vi "Begin.vi"(8 "error in":errorcluster, 11 "HARDWARE cluster":T7={"DRIVE MOTORS"=[], "Controller"=[], "ENCODERS"=[], "GYRO HARDWARE"={"Descr"="GYRO", "Installed?"=FALSE, "SPI Bus"=enum."SPI On-Board, CS0", "AnalogChannel"=enum."AI 0", "Calibrate On Open"=TRUE, "Calibrated Center Voltage"=0.0, "Calibration Time (s)"=2.0, "Sample Rate (Hz)"=100.0, "RefName"="", "stack name"="GYRO"}, "AIR"={"PRESSURE"=[], "COMPRESSOR"={"Descr"="COMPRESSOR", "Installed?"=TRUE, "Pneumatics Control Module"=0, "RefName"="COMPRESSOR", "stack name"="COMPRESSOR"}, "SOLENOIDS"=[]}, "MOTORS"=[], "SERVOS"=[], "SONAR"=[], "RELAY"=[], "LIMIT"=[]} {"MOTORS"."CAN ID" min=1 max=62 step=1; "MOTORS"."Motor Controller" items=["SPARK", "Existing", "SD540", "TALON SRX", "VICTOR SP", "TALON SR", "JAGUAR", "VICTOR"]; "AIR"."PRESSURE"."warning HIGH" format="%.2f"; "AIR"."PRESSURE"."warning LOW" format="%.2f"; "AIR"."PRESSURE"."nominal value" format="%.2f"; "DRIVE MOTORS"."CAN ID" min=1 max=62 step=1; "DRIVE MOTORS"."Motor Controller" items=["SPARK", "Existing", "SD540", "TALON SRX", "VICTOR SP", "TALON SR", "JAGUAR", "VICTOR"]; "Controller"."Parameters"."DEADBAND" format="%#_13g"; "Controller"."Parameters"."MIN SPEED" format="%#_13g"; "Controller"."Parameters"."MAX LIMIT" format="%#_13g"}) -> (0 "error out":errorcluster)   [LabVIEW 2019]
doc: "Called before other user functions, this VI is expected to open initial I/O refnums, load in file data, and do all program initialization. Notice that the <B>error out</B> terminal is simply used for data flow. Wiring it to other structures or subVIs ensures that this VI runs first."
uses:
  Controls/def HARDWARE CTRL info.ctl
  Controls/def MOTOR info.ctl
  Controls/ctrl MOTOR CTRLR SELECT.ctl
  <vilib>/Rock Robotics/SystemInterfaces/DIO/FPGA_DIOPWMChannel.ctl
  <vilib>/Rock Robotics/WPI/ThirdParty/REV Robotics/SPARK MAX/Typedef/Spark MAX Motor Type.ctl
  Controls/def USER CONTROL info.ctl
  <vilib>/Rock Robotics/WPI/Joystick/WPI_JoystickDeviceEnum.ctl
  Controls/def JOYSTICK PARAMETERS.ctl
  Controls/def ENCODER info.ctl
  <vilib>/Rock Robotics/SystemInterfaces/DIO/FPGA_DIOChannel.ctl
  <vilib>/Rock Robotics/WPI/Encoder/WPI_EncoderType.ctl
  Controls/def GYRO info.ctl
  <vilib>/Rock Robotics/SystemInterfaces/spilib/spi_bus.ctl
  Controls/ctrl ANALOG CHANNEL SELECT.ctl
  Controls/def AIR PRESSURE info.ctl
  <vilib>/Rock Robotics/SystemInterfaces/AI/FPGA_AIChannel.ctl
  Controls/def COMPRESSOR info.ctl
  Controls/def SOLENOID info.ctl
  <vilib>/Rock Robotics/WPI/Solenoid/WPI_SolenoidChannel.ctl
  <vilib>/Rock Robotics/WPI/Solenoid/WPI_SolenoidValue.ctl
  Controls/def SERVO info.ctl
  Controls/def SONAR info.ctl
  Controls/ctrl SONAR DEVICE SELECT.ctl
  <vilib>/Rock Robotics/WPI/Ultrasonic/WPI_UltrasonicRangeUnits.ctl
  Controls/def RELAY info.ctl
  <vilib>/Rock Robotics/SystemInterfaces/DIO/FPGA_DIORelayChannel.ctl
  <vilib>/Rock Robotics/WPI/Relay/WPI_RelayDirection.ctl
  <vilib>/Rock Robotics/WPI/Relay/WPI_RelayValue.ctl
  Controls/def LIMIT SWITCH info.ctl
  <vilib>/Rock Robotics/WPI/RobotDrive/WPI_RobotDriveDevRef.ctl
  <vilib>/Rock Robotics/WPI/MotorControl/WPI_MotorControlDeviceRef.ctl
  <vilib>/Rock Robotics/WPI/MotorControl/WPI_MotorControlType.ctl
  <vilib>/Rock Robotics/WPI/PWM/WPI_PWMDeadband.ctl
  <vilib>/Rock Robotics/WPI/DriverStation/WPI_DriverStationRobotMode2.ctl
  <vilib>/Rock Robotics/WPI/SafetyOutput/WPI_SafetyOutputConfigMenu.ctl
  Robot Global Data.vi
  <vilib>/Rock Robotics/WPI/Switch/WPI_SwitchOpenLimit.vi
  <vilib>/Rock Robotics/WPI/Solenoid/WPI_SolenoidOpenDouble.vi
  <vilib>/Rock Robotics/WPI/Solenoid/WPI_SolenoidOpenSingle.vi
  <vilib>/Rock Robotics/WPI/Solenoid/WPI_SolenoidSetEnum.vi
  <vilib>/Rock Robotics/WPI/Utilities/WPI_GetSetVariantRefNum.vi
  <vilib>/Rock Robotics/WPI/Counter/WPI_CounterDigitalInputToDigitalSource.vi
  <vilib>/Rock Robotics/WPI/MotorControl/WPI_MotorControlOpen SPARK.vi
  <vilib>/Rock Robotics/WPI/MotorControl/WPI_MotorControlOpen SD540.vi
  <vilib>/Rock Robotics/WPI/MotorControl/WPI_MotorControlOpen TalonSRX.vi
  <vilib>/Rock Robotics/WPI/MotorControl/WPI_MotorControlOpen VictorSP.vi
  <vilib>/Rock Robotics/WPI/MotorControl/WPI_MotorControlOpen Talon.vi
  <vilib>/Rock Robotics/WPI/MotorControl/WPI_MotorControlOpen Jaguar.vi
  <vilib>/Rock Robotics/WPI/MotorControl/WPI_MotorControlOpen Victor.vi
  Global  HARDWARE.vi
  <vilib>/Rock Robotics/WPI/Ultrasonic/WPI_SonarSRF08DeviceAddress.ctl
  <vilib>/Rock Robotics/SystemInterfaces/i2clib/i2c_bus.ctl
  <vilib>/Rock Robotics/WPI/Ultrasonic/WPI_SonarSRF04DigitalOpen.vi
  <vilib>/Rock Robotics/WPI/Ultrasonic/WPI_SonarSRF04DigitalRefNum Registry Set.vi
  <vilib>/Rock Robotics/WPI/Gyro/WPI_GyroAnalogOpen.vi
panel:
  out "RobotDriveDevRef":T1={"DevStatus"={"status"=FALSE, "code"=0, "source"=""}, "Motors[]"=[], "Square Inputs"=FALSE, "Max Output"=1.0}
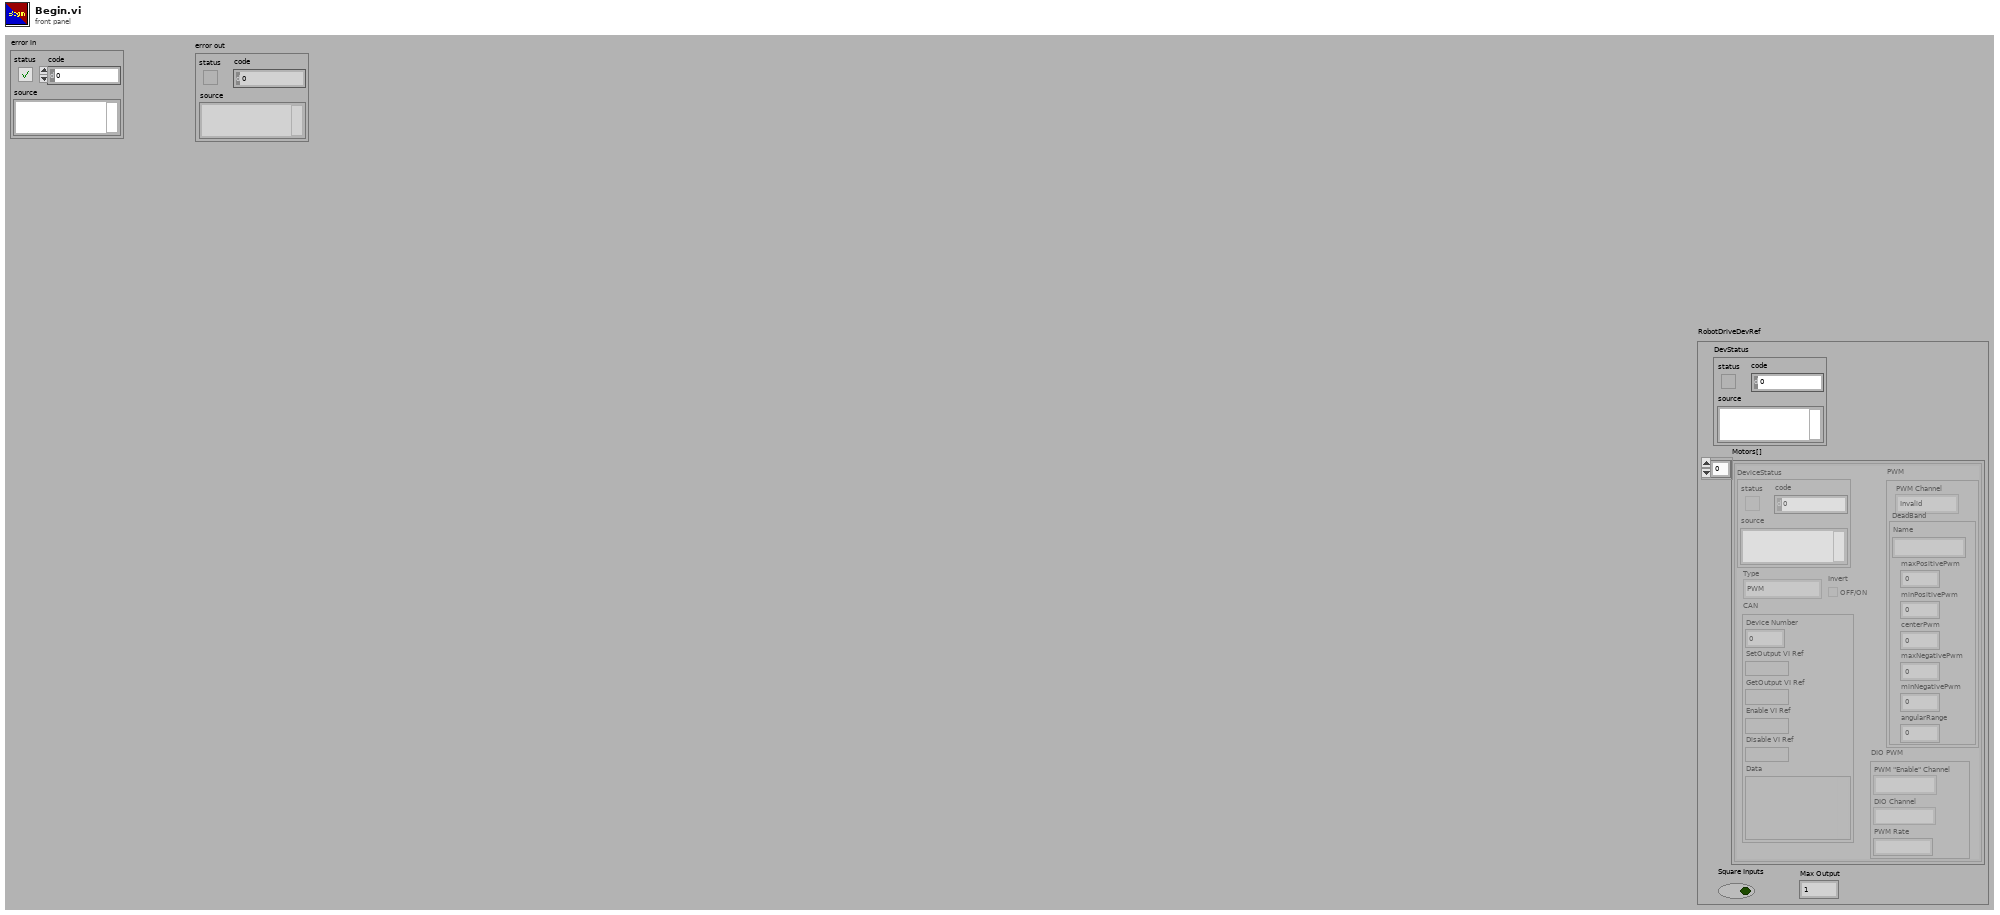
[diagram p1: front panel]
types:
  T1 = typedef "WPI_RobotDriveDevRef.ctl" = cluster{"DevStatus":errorcluster, "Motors[]":T2[], "Square Inputs":bool, "Max Output":dbl}
  T2 = typedef "WPI_MotorControlDeviceRef.ctl" = cluster{"DeviceStatus":errorcluster, "Type":T3, "PWM":cluster{"PWM Channel":T4, "DeadBand":T5}, "CAN":cluster{"Device Number":u8, "SetOutput VI Ref":variant, "GetOutput VI Ref":variant, "Enable VI Ref":variant, "Disable VI Ref":variant, "Data":variant}, "Invert":bool, "DIO PWM":cluster{"PWM \"Enable\" Channel":T4, "DIOChannel":T6, "PWM Rate":dbl}}
  T3 = typedef "WPI_MotorControlType.ctl" = enum16{"PWM", "CAN", "DIO PWM"}
  T4 = typedef "FPGA_DIOPWMChannel.ctl" = enum8{"PWM 0", "PWM 1", "PWM 2", "PWM 3", "PWM 4", "PWM 5", "PWM 6", "PWM 7", "PWM 8", "PWM 9", "PWM MXP 0", "PWM MXP 1", "PWM MXP 2", "PWM MXP 3", "PWM MXP 4", "PWM MXP 5", "PWM MXP 6", "PWM MXP 7", "PWM MXP 8", "PWM MXP 9", "Invalid"}
  T5 = typedef "WPI_PWMDeadband.ctl" = cluster{"Name":string, "maxPositivePwm":i32, "minPositivePwm":i32, "centerPwm":i32, "maxNegativePwm":i32, "minNegativePwm":i32, "angularRange":u16}
  T6 = typedef "FPGA_DIOChannel.ctl" = enum8{"DIO 0", "DIO 1", "DIO 2", "DIO 3", "DIO 4", "DIO 5", "DIO 6", "DIO 7", "DIO 8", "DIO 9", "DIO MXP 0", "DIO MXP 1", "DIO MXP 2", "DIO MXP 3", "DIO MXP 4", "DIO MXP 5", "DIO MXP 6", "DIO MXP 7", "DIO MXP 8", "DIO MXP 9", "DIO MXP 10", "DIO MXP 11", "DIO MXP 12", "DIO MXP 13", "DIO MXP 14", "DIO MXP 15", "SPI Port CS1", "SPI Port CS2", "SPI Port CS3", "SPI Port MISO", "SPI Port MOSI", "Invalid"}
  T7 = typedef "def HARDWARE CTRL info.ctl" = cluster{"DRIVE MOTORS":T8[], "Controller":T11[], "ENCODERS":T14[], "GYRO HARDWARE":T16, "AIR":cluster{"PRESSURE":T19[], "COMPRESSOR":T21, "SOLENOIDS":T22[]}, "MOTORS":T8[], "SERVOS":T25[], "SONAR":T26[], "RELAY":T29[], "LIMIT":T33[]}
  T8 = typedef "def MOTOR info.ctl" = cluster{"Descr":string, "Motor Controller":T9, "PWM ch":T4, "Invert?":bool, "Installed?":bool, "RefName":string, "stack name":string, "remove deadband":bool, "CAN ID":u8, "IDLE BEHAVIOUR":string, "Motor Type":T10}
  T9 = typedef "ctrl MOTOR CTRLR SELECT.ctl" = u16
  T10 = typedef "Spark MAX Motor Type.ctl" = enum16{"Brushed", "Brushless"}
  T11 = typedef "def USER CONTROL info.ctl" = cluster{"Descr":string, "Installed?":bool, "RefName":string, "JoystickDevice":T12, "Invert Y axis":bool, "Scale":dbl, "AXIS":string, "BUTTONS":string, "POV":string, "Parameters":T13}
  T12 = typedef "WPI_JoystickDeviceEnum.ctl" = enum16{"USB 0", "USB 1", "USB 2", "USB 3", "USB 4", "USB 5"}
  T13 = typedef "def JOYSTICK PARAMETERS.ctl" = cluster{"MAX LIMIT":dbl, "MIN SPEED":dbl, "DEADBAND":dbl, "invert X?":bool, "invert Y?":bool}
  T14 = typedef "def ENCODER info.ctl" = cluster{"Descr":string, "Installed?":bool, "A Channel":T6, "B Channel":T6, "Invert Direction":bool, "Enum":T15, "Gear ratio":dbl, "Cycles per Rev":dbl, "Diameter (in)":dbl[unit], "RefName":string, "stack name":string, "min rate (hz)":dbl, "Samples":u8, "STACK subnames":cluster{"RESET name":string, "STOPPED name":string, "DIRECTION name":string, "RATE name":string, "INSTALLED name":string}}
  T15 = typedef "WPI_EncoderType.ctl" = enum16{"1x", "2x", "4x"}
  T16 = typedef "def GYRO info.ctl" = cluster{"Descr":string, "Installed?":bool, "SPI Bus":T17, "AnalogChannel":T18, "Calibrate On Open":bool, "Calibrated Center Voltage":dbl, "Calibration Time (s)":dbl, "Sample Rate (Hz)":dbl, "RefName":string, "stack name":string}
  T17 = typedef "spi_bus.ctl" = enum16{"SPI On-Board, CS0", "SPI On-Board, CS1", "SPI On-Board, CS2", "SPI On-Board, CS3", "SPI MXP", "Invalid"}
  T18 = typedef "ctrl ANALOG CHANNEL SELECT.ctl" = enum8{"AI 0", "AI 1", "Invalid"}
  T19 = typedef "def AIR PRESSURE info.ctl" = cluster{"Descr":string, "Installed?":bool, "Channel":T20, "RefName":string, "stack name":string, "MULTIPLIER":dbl, "OFFSET":dbl, "nominal value":dbl, "warning LOW":dbl, "warning HIGH":dbl}
  T20 = typedef "FPGA_AIChannel.ctl" = enum8{"AI 0", "AI 1", "AI 2", "AI 3", "AI MXP 0", "AI MXP 1", "AI MXP 2", "AI MXP 3", "Invalid"}
  T21 = typedef "def COMPRESSOR info.ctl" = cluster{"Descr":string, "Installed?":bool, "Pneumatics Control Module":u8, "RefName":string, "stack name":string}
  T22 = typedef "def SOLENOID info.ctl" = cluster{"Descr":string, "Installed?":bool, "Pneumatics Control Module (0)":u8, "DBL":bool, "SolenoidChannel":T23, "SolenoidChannel":T23, "Default SET":T24, "RefName":string, "Value":string}
  T23 = typedef "WPI_SolenoidChannel.ctl" = enum8{"Solenoid 0", "Solenoid 1", "Solenoid 2", "Solenoid 3", "Solenoid 4", "Solenoid 5", "Solenoid 6", "Solenoid 7", "Invalid"}
  T24 = typedef "WPI_SolenoidValue.ctl" = enum16{"Off", "On", "Forward", "Reverse"}
  T25 = typedef "def SERVO info.ctl" = cluster{"Descr":string, "PWM ch":T4, "Installed?":bool, "Angular range":dbl, "RefName":string, "stack name":string}
  T26 = typedef "def SONAR info.ctl" = cluster{"Descr":string, "Installed?":bool, "Device type":T27, "PING Channel":T6, "ECHO Channel":T6, "RefName":string, "stack name":string, "Samples":i32, "Range Units":T28}
  T27 = typedef "ctrl SONAR DEVICE SELECT.ctl" = enum16{"SRF04 Digital", "MB1010 Digital", "MB1010 Analog", "SRF08 Digital"}
  T28 = typedef "WPI_UltrasonicRangeUnits.ctl" = enum16{"inches", "mm"}
  T29 = typedef "def RELAY info.ctl" = cluster{"Descr":string, "Installed?":bool, "RelayChannel":T30, "Relay Direction":T31, "Relay Value":T32, "RefName":string, "Value":string}
  T30 = typedef "FPGA_DIORelayChannel.ctl" = enum8{"Relay 0", "Relay 1", "Relay 2", "Relay 3", "Invalid"}
  T31 = typedef "WPI_RelayDirection.ctl" = enum16{"Both directions", "Forward only", "Reverse only"}
  T32 = typedef "WPI_RelayValue.ctl" = enum16{"Off", "On", "Forward", "Reverse"}
  T33 = typedef "def LIMIT SWITCH info.ctl" = cluster{"Descr":string, "Installed?":bool, "A Channel":T6, "Normally Closed?":bool, "RefName":string, "stack name":string}
  T34 = typedef "WPI_DriverStationRobotMode2.ctl" = enum16{"Autonomous Disabled", "Autonomous Enabled", "Teleop Disabled", "Teleop Enabled", "Disconnected", "Finish", "Test Disabled", "Test Enabled", "Emergency Stopped"}
  T35 = cluster{"PRESSURE":T19[], "COMPRESSOR":T21, "SOLENOIDS":T22[]}
  T36 = typedef "WPI_AnalogChannelDevRef.ctl" = cluster{"DevStatus":errorcluster, "Analog Channel":T20}
  T37 = typedef "WPI_SolenoidDevRef.ctl" = cluster{"DevStatus":errorcluster, "Pneumatics Control Module":u8, "Forward Solenoid Channel":T23, "Reverse Solenoid Channel":T23}
  T38 = typedef "WPI_CompressorDevRef.ctl" = cluster{"DevStatus":errorcluster, "Pneumatics Control Module":u8}
  T39 = typedef "WPI_RelayDevRef.ctl" = cluster{"DevStatus":errorcluster, "Relay Channel":T30, "Relay Direction":T31}
  T40 = typedef "WPI_SwitchDevRef.ctl" = cluster{"DevStatus":errorcluster, "DIO Channel":T6, "CntIndex":T41, "Normally Closed":bool}
  T41 = typedef "FPGA_CounterCtrSystemIndex.ctl" = enum8{"Ctr 0", "Ctr 1", "Ctr 2", "Ctr 3", "Ctr 4", "Ctr 5", "Ctr 6", "Ctr 7", "Invalid"}
  T42 = typedef "i2c_bus.ctl" = enum16{"I2C On-Board", "I2C MXP", "Invalid"}
  T43 = typedef "WPI_UltrasonicDeviceRef.ctl" = cluster{"DevStatus":errorcluster, "Ping Channel":T6, "Echo Channel":T6, "CntIndex":T41}
  T44 = typedef "WPI_SonarSRF08DeviceAddress.ctl" = u8
  T45 = typedef "WPI_ServoDeviceRef.ctl" = cluster{"DeviceStatus":errorcluster, "PWM Channel":T4, "DeadBand":T5}
  T46 = typedef "WPI_GyroDevRef.ctl" = cluster{"DevStatus":errorcluster, "Analog Channel":T20, "Gain (VoltsPerDegree/Second)":dbl, "Gyro Type":enum16{"Analog", "XRS450"}, "Handle":i32, "SPI Bus":T17, "Device Found":bool, "Sample Rate":dbl, "Calibrate On Open":bool, "Offset":dbl}
  T47 = typedef "WPI_JoystickDevRef.ctl" = cluster{"Device":T12}
  T48 = typedef "WPI_SafetyOutputConfigMenu.ctl" = enum16{"Enable", "Disable"}
  T49 = typedef "WPI_DigitalInputDevRef.ctl" = cluster{"DevStatus":errorcluster, "DIO Channel":T6}
  T50 = typedef "FPGA_CounterEncoderSourceConvertionLVSourceType.ctl" = cluster{"DevStatus":errorcluster, "AnalogTriggerMode?":bool, "DigitalMode":cluster{"DIO Channel":T51}, "AnalogTriggerMode":cluster{"AnalogTriggerIndex":T52, "OutputType":T53}}
  T51 = typedef "FPGA_DIODigitalSourceChannel.ctl" = enum8{"DIO 0", "DIO 1", "DIO 2", "DIO 3", "DIO 4", "DIO 5", "DIO 6", "DIO 7", "DIO 8", "DIO 9", "DIO MXP 0", "DIO MXP 1", "DIO MXP 2", "DIO MXP 3", "DIO MXP 4", "DIO MXP 5", "DIO MXP 6", "DIO MXP 7", "DIO MXP 8", "DIO MXP 9", "DIO MXP 10", "DIO MXP 11", "DIO MXP 12", "DIO MXP 13", "DIO MXP 14", "DIO MXP 15", "SPI Port CS1", "SPI Port CS2", "SPI Port CS3", "SPI Port MISO", "SPI Port MOSI", "Disabled"}
  T52 = typedef "FPGA_AnalogTriggerIndex.ctl" = enum8{"Trig 0", "Trig 1", "Trig 2", "Trig 3", "Trig 4", "Trig 5", "Trig 6", "Trig 7", "Invalid"}
  T53 = typedef "FPGA_AnalogTriggerOutType.ctl" = enum16{"InWindow", "TriggerState", "Rising", "Falling"}
  T54 = typedef "WPI_EncoderDevRef.ctl" = cluster{"DevStatus":errorcluster, "EncoderIndex":T55, "CounterIndex":T41, "DistancePerCount":dbl, "Decoding Type":T15}
  T55 = typedef "FPGA_EncoderIdx.ctl" = enum8{"Enc 0", "Enc 1", "Enc 2", "Enc 3", "Enc 4", "Enc 5", "Enc 6", "Enc 7", "Invalid"}
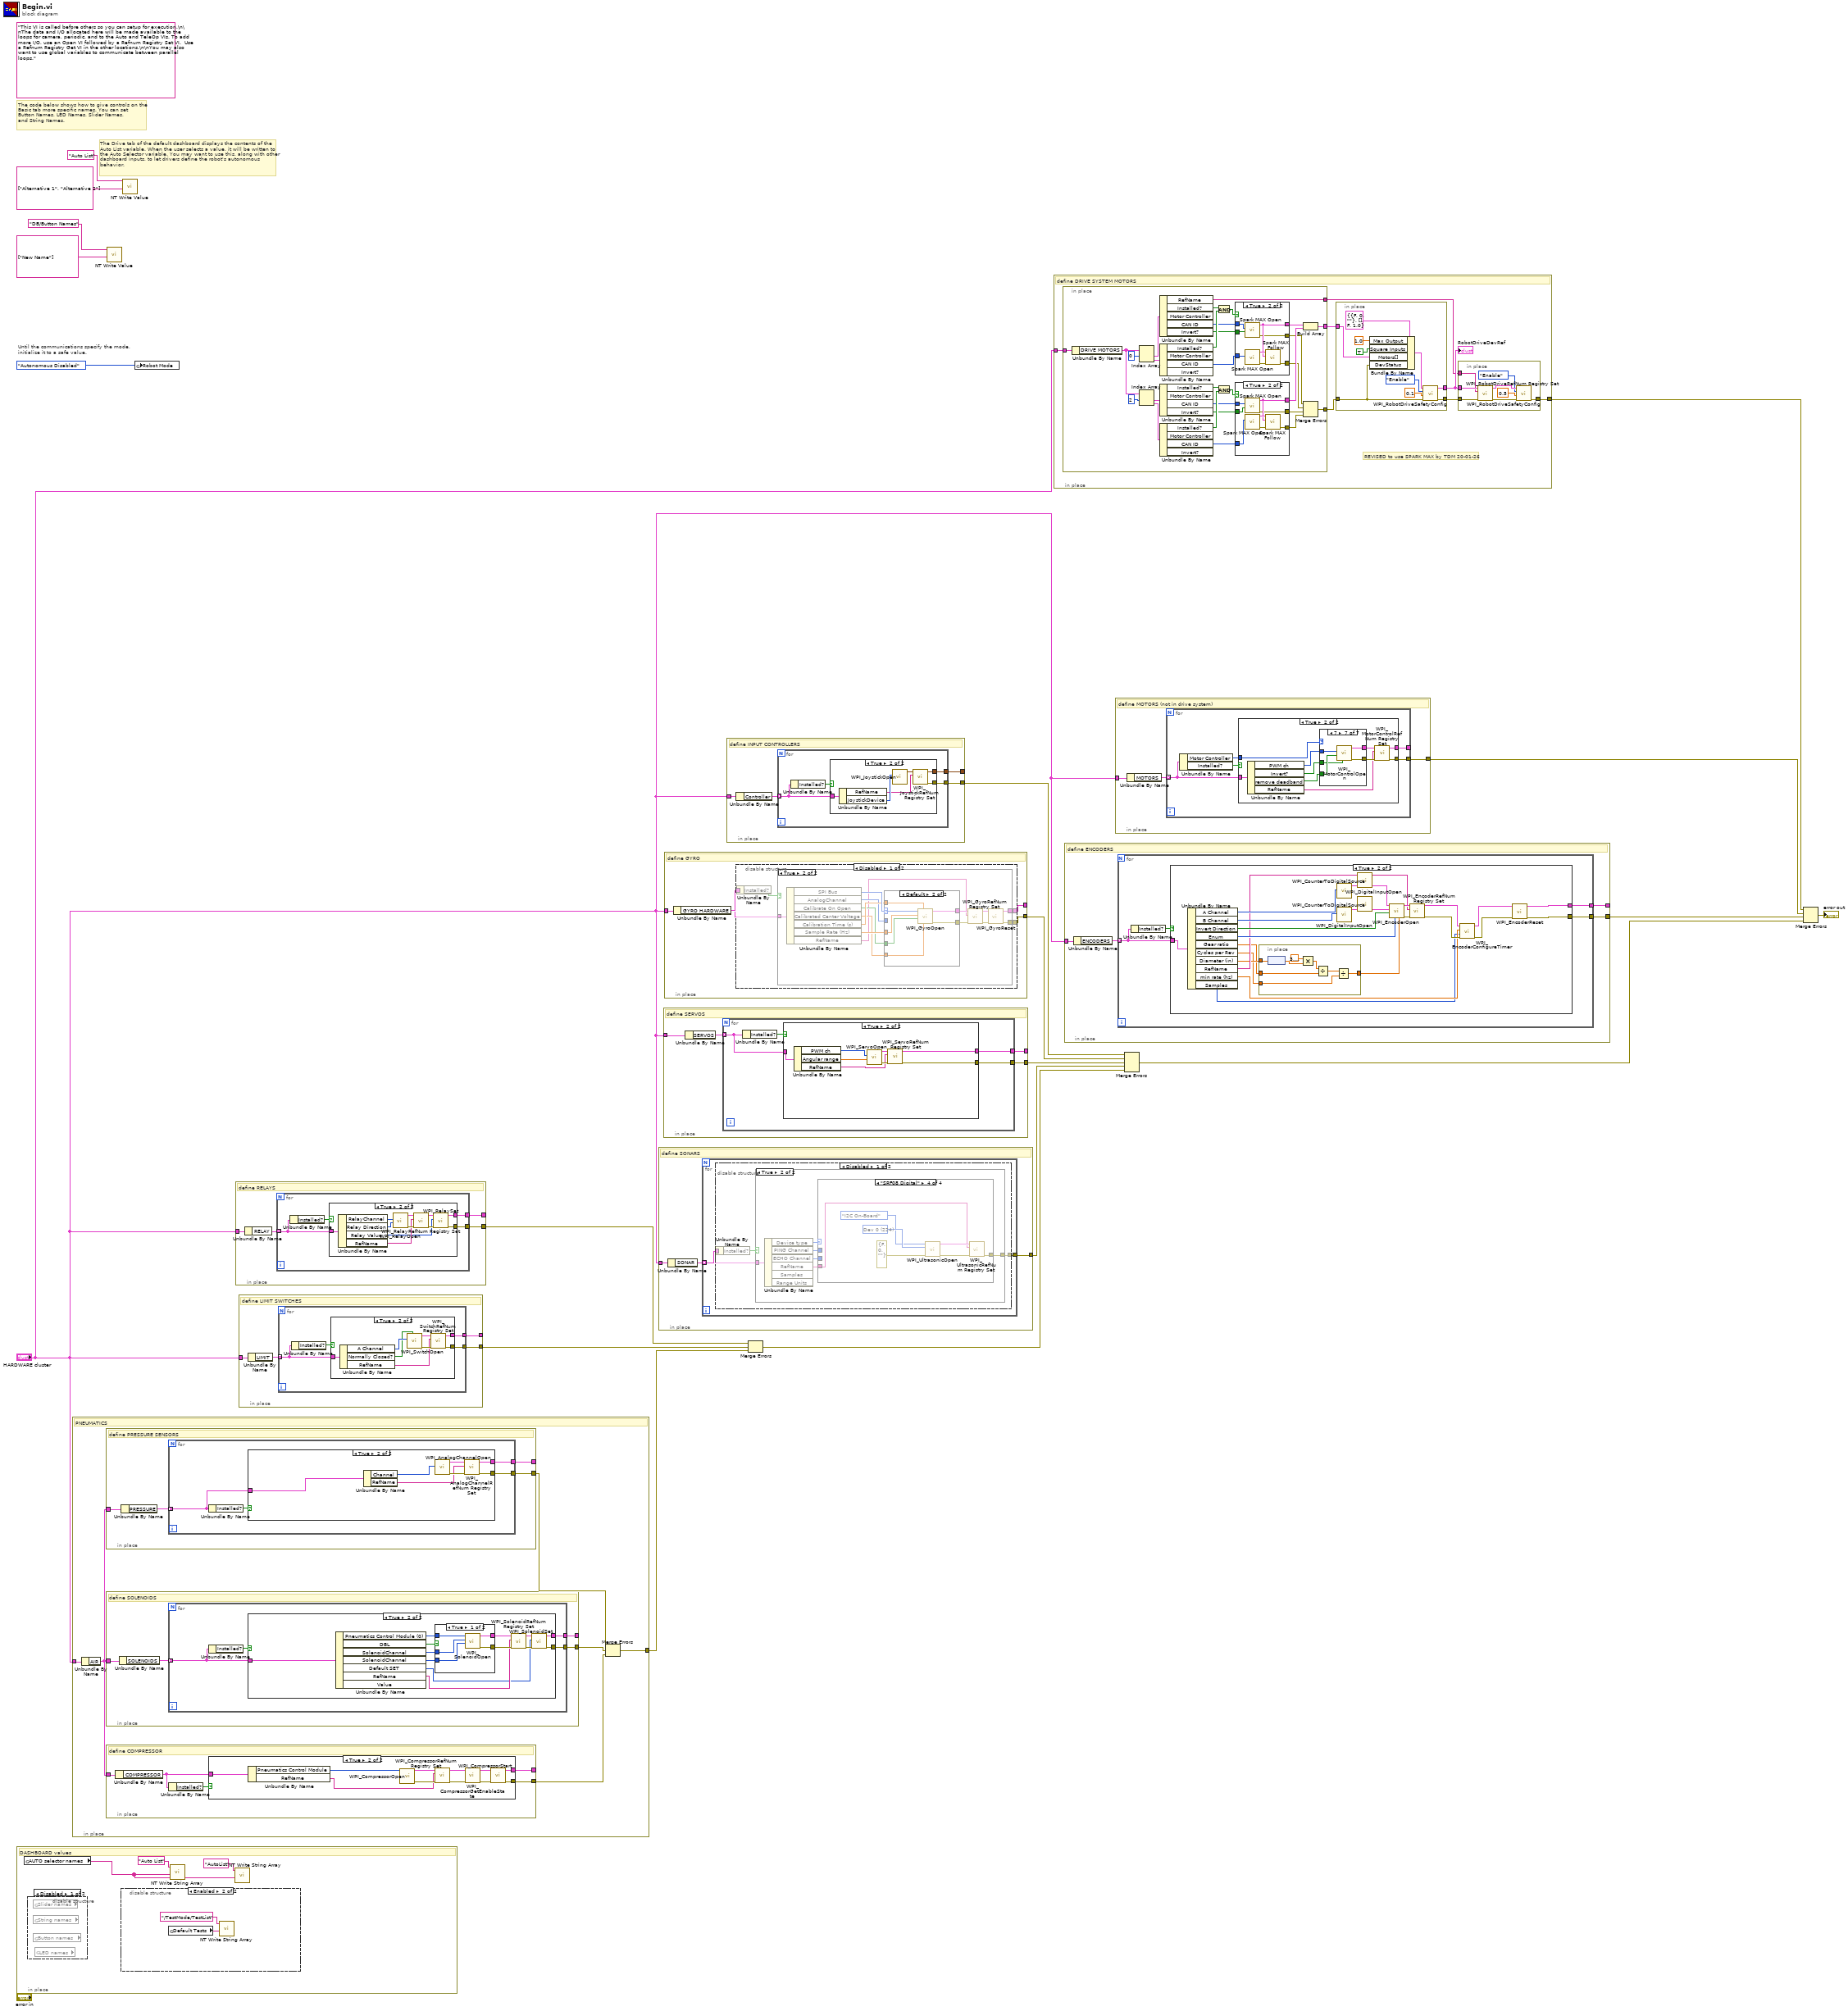
[diagram p0: block diagram]
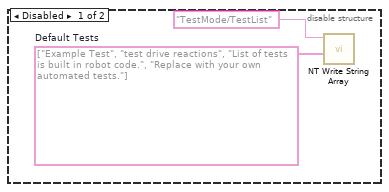
[diagram p2: hidden frame]
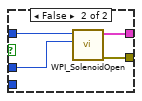
[diagram p6: hidden frame]
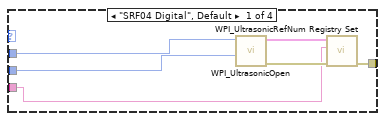
[diagram p11: hidden frame]
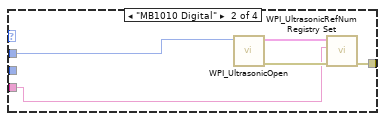
[diagram p12: hidden frame]
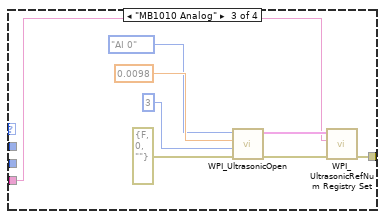
[diagram p13: hidden frame]
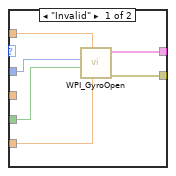
[diagram p17: hidden frame]
diagram:
  (unwired) "This VI is called before others so you can setup for execution.\n\nThe data and I/O allocated here will be made available to the loops for camera, periodic, and to the Auto and TeleOp VIs. To add more I/O, use an Open VI followed by a Refnum Registry Set VI.  Use a Refnum Registry Get VI in the other locations.\n\nYou may also want to use global variables to communicate between parallel loops."
  # "The Drive tab of the default dashboard displays the contents of the\nAuto List variable. When the user selects a value, it will be written to\nthe Auto Selector variable. You may want to use this, along with other\ndashboard inputs, to let drivers define the robot's autonomous\nbehavior."
  # "The code below shows how to give controls on the\nBasic tab more specific names. You can set\nButton Names, LED Names, Slider Names,\nand String Names."
  # "Until the communications specify the mode,\ninitialize it to a safe value."
  n1 = in-place {
    # "DASHBOARD values"
    n2 = global read "Global  HARDWARE.vi" "AUTO selector names"() -> (w20:string[])
    n3 = disable-structure shown="Disabled" {
      frame Disabled {
        n4 = global read "Global  HARDWARE.vi" "Slider names"() -> ()  [unwired: 1 out]
        n5 = global read "Global  HARDWARE.vi" "String names"() -> ()  [unwired: 1 out]
        n6 = global read "Global  HARDWARE.vi" "Button names"() -> ()  [unwired: 1 out]
        n7 = global read "Global  HARDWARE.vi" "LED names"() -> ()  [unwired: 1 out]
      }
      frame Enabled {
      }
    }
    n8 = disable-structure shown="Enabled" {
      frame Disabled {
        w24 = string[] ["Example Test", "test drive reactions", "List of tests is built in robot code.", "Replace with your own automated tests."]  # Default Tests
        n9 = call <vilib>:"NT Write String Array.vi"("String Array"=w24, "Name"="TestMode/TestList") -> ()  [unwired: 9 in, 1 out]
      }
      frame Enabled {
        n10 = global read "Global  HARDWARE.vi" "Default Tests"() -> (w26:string[])
        n11 = call <vilib>:"NT Write String Array.vi"("String Array"=w26, "Name"="/TestMode/TestList") -> ()  [unwired: 9 in, 1 out]
      }
    }
    n12 = call <vilib>:"NT Write String Array.vi"("String Array"=w20, "Name"="Auto List") -> ()  [unwired: 9 in, 1 out]
    n13 = call <vilib>:"NT Write String Array.vi"("String Array"=w20, "Name"="AutoList") -> ()  [unwired: 9 in, 1 out]
  }
  n14 = in-place {
    in-place-border: "HARDWARE cluster" -> [w32]
    in-place-border: [w27] -> w3
    # "PNEUMATICS"
    n15 = Unbundle By Name(w32) -> ("AIR"=w31:T35)
    n16 = in-place {
      in-place-border: w31 -> [w36]
      in-place-border: [w34] -> _
      in-place-border: [w33] -> w28
      # "define PRESSURE SENSORS"
      n17 = Unbundle By Name(w36) -> ("PRESSURE"=w35:T19[])
      n18 = for {
        tunnel: w35 -> [w39] mode=indexing
        tunnel: [w38] -> w34
        tunnel: [w37] -> w33
        n19 = Unbundle By Name(w39) -> ("Installed?"=w40:bool)
        n20 = case shown="True" w40 {
          tunnel: w39 -> [_ w47]
          tunnel: [_ w42] -> w38
          tunnel: [_ w41] -> w37
          frame False {
          }
          frame True {
            n21 = Unbundle By Name(w47) -> ("Channel"=w44:T20, "RefName"=w43:string)
            n22 = call <vilib>:"WPI_AnalogChannelOpen.vi"("Analog Channel"=w44) -> ("error out"=w45:errorcluster, "AIDeviceRef"=w46:T36)  [unwired: 9 in]
            n23 = call <vilib>:"WPI_AnalogChannelRefNum Registry Set.vi"("error in (no error)"=w45, "refnum name"=w43, "AIDeviceRef"=w46) -> ("error out"=w41:errorcluster, "AIDeviceRef"=w42:T36)  [unwired: 7 in]
          }
        }
      }
    }
    n24 = in-place {
      in-place-border: w31 -> [w51]
      in-place-border: [w49] -> _
      in-place-border: [w48] -> w29
      # "define SOLENOIDS"
      n25 = Unbundle By Name(w51) -> ("SOLENOIDS"=w50:T22[])
      n26 = for {
        tunnel: w50 -> [w54] mode=indexing
        tunnel: [w53] -> w49
        tunnel: [w52] -> w48
        n27 = Unbundle By Name(w54) -> ("Installed?"=w55:bool)
        n28 = case shown="True" w55 {
          tunnel: w54 -> [_ w68]
          tunnel: [_ w57] -> w53
          tunnel: [_ w56] -> w52
          frame False {
          }
          frame True {
            n29 = Unbundle By Name(w68) -> ("Pneumatics Control Module (0)"=w67:u8, "DBL"=w66:bool, "SolenoidChannel"=w65:T23, "SolenoidChannel"=w64:T23, "Default SET"=w58:T24, "RefName"=w62:string)  [unwired: 1 out]
            n30 = case shown="True" w66 {
              tunnel: w67 -> [w73 w77]
              tunnel: w65 -> [w72 w76]
              tunnel: w64 -> [w71 _]
              tunnel: [w70 w75] -> w61
              tunnel: [w69 w74] -> w63
              frame True {
                n31 = call-poly <vilib>:"WPI_SolenoidOpen.vi"("Reverse Solenoid Channel"=w71, "Forward Solenoid Channel"=w72, "Pneumatics Control Module (0)"=w73) -> ("error out"=w69:errorcluster, "SolenoidDevRef"=w70:T37)  [unwired: 7 in]
              }
              frame False {
                n32 = call-poly <vilib>:"WPI_SolenoidOpen.vi"("Solenoid Channel"=w76, "Pneumatics Control Module (0)"=w77) -> ("error out"=w74:errorcluster, "SolenoidDevRef"=w75:T37)  [unwired: 8 in]
              }
            }
            n33 = call <vilib>:"WPI_SolenoidRefNum Registry Set.vi"("error in (no error)"=w63, "refnum name"=w62, "SolenoidDevRef"=w61) -> ("error out"=w60:errorcluster, "SolenoidDevRef"=w59:T37)  [unwired: 7 in]
            n34 = call-poly <vilib>:"WPI_SolenoidSet.vi"("error in (no error)"=w60, "Value"=w58, "SolenoidDevRef"=w59) -> ("error out"=w56:errorcluster, "SolenoidDevRef"=w57:T37)  [unwired: 7 in]
          }
        }
      }
    }
    n35 = in-place {
      in-place-border: w31 -> [w82]
      in-place-border: [w79] -> _
      in-place-border: [w78] -> w30
      # "define COMPRESSOR"
      n36 = Unbundle By Name(w82) -> ("COMPRESSOR"=w80:T21)
      n37 = Unbundle By Name(w80) -> ("Installed?"=w81:bool)
      n38 = case shown="True" w81 {
        tunnel: w80 -> [_ w91]
        tunnel: [_ w84] -> w79
        tunnel: [_ w83] -> w78
        frame False {
        }
        frame True {
          n39 = Unbundle By Name(w91) -> ("Pneumatics Control Module"=w90:u8, "RefName"=w89:string)
          n40 = call <vilib>:"WPI_CompressorOpen.vi"("Pneumatics Control Module (0)"=w90) -> ("CompressorDevRef"=w92:T38, "error out"=w93:errorcluster)  [unwired: 13 in]
          n41 = call <vilib>:"WPI_CompressorRefNum Registry Set.vi"("error in (no error)"=w93, "refnum name"=w89, "CompressorDevRef"=w92) -> ("error out"=w88:errorcluster, "CompressorDevRef"=w87:T38)  [unwired: 7 in]
          n42 = call <vilib>:"WPI_CompressorGetEnableState.vi"("error in (no error)"=w88, "CompressorDevRef"=w87) -> ("error out"=w86:errorcluster, "CompressorDevRef"=w85:T38)  [unwired: 6 in, 2 out]
          n43 = call <vilib>:"WPI_CompressorStart.vi"("error in (no error)"=w86, "CompressorDevRef"=w85) -> ("error out"=w83:errorcluster, "CompressorDevRef"=w84:T38)  [unwired: 8 in]
        }
      }
    }
    n44 = Merge Errors(w28, w29, w30) -> (w27:errorcluster)
  }
  n45 = call-poly <vilib>:"NT Write Value.vi"("String Array"=string[] ["New Name"], "Name"="DB/Button Names") -> ()  [unwired: 9 in, 1 out]
  n46 = call-poly <vilib>:"NT Write Value.vi"("String Array"=string[] ["Alternative 1", "Alternative 2"], "Name"="Auto List") -> ()  [unwired: 9 in, 1 out]
  n47 = global write "Robot Global Data.vi" "Robot Mode"(WPI_DriverStationRobotMode2."Autonomous Disabled" ("Robot Mode")) -> ()
  n48 = in-place {
    in-place-border: "HARDWARE cluster" -> [w97]
    in-place-border: [w95] -> _
    in-place-border: [w94] -> w13
    # "define RELAYS"
    n49 = Unbundle By Name(w97) -> ("RELAY"=w96:T29[])
    n50 = for {
      tunnel: w96 -> [w100] mode=indexing
      tunnel: [w99] -> w95
      tunnel: [w98] -> w94
      n51 = Unbundle By Name(w100) -> ("Installed?"=w101:bool)
      n52 = case shown="True" w101 {
        tunnel: w100 -> [_ w110]
        tunnel: [_ w103] -> w99
        tunnel: [_ w102] -> w98
        frame False {
        }
        frame True {
          n53 = Unbundle By Name(w110) -> ("RelayChannel"=w109:T30, "Relay Direction"=w108:T31, "Relay Value"=w104:T32, "RefName"=w107:string)
          n54 = call <vilib>:"WPI_RelayOpen.vi"("Relay Direction"=w108, "Relay Channel"=w109) -> ("error out"=w112:errorcluster, "RelayDevRef"=w111:T39)  [unwired: 8 in]
          n55 = call <vilib>:"WPI_RelayRefNum Registry Set.vi"("error in (no error)"=w112, "refnum name"=w107, "RelayDevRef"=w111) -> ("error out"=w106:errorcluster, "RelayDevRef"=w105:T39)  [unwired: 7 in]
          n56 = call <vilib>:"WPI_RelaySet.vi"("error in (no error)"=w106, "RelayValue"=w104, "RelayDevRef"=w105) -> ("error out"=w102:errorcluster, "RelayDevRef"=w103:T39)  [unwired: 7 in]
        }
      }
    }
  }
  n57 = in-place {
    in-place-border: "HARDWARE cluster" -> [w116]
    in-place-border: [w114] -> _
    in-place-border: [w113] -> w12
    # "define LIMIT SWITCHES"
    n58 = Unbundle By Name(w116) -> ("LIMIT"=w115:T33[])
    n59 = for {
      tunnel: w115 -> [w119] mode=indexing
      tunnel: [w118] -> w114
      tunnel: [w117] -> w113
      n60 = Unbundle By Name(w119) -> ("Installed?"=w120:bool)
      n61 = case shown="True" w120 {
        tunnel: w119 -> [_ w128]
        tunnel: [_ w122] -> w118
        tunnel: [_ w121] -> w117
        frame False {
        }
        frame True {
          n62 = Unbundle By Name(w128) -> ("A Channel"=w127:T6, "Normally Closed?"=w126:bool, "RefName"=w123:string)
          n63 = call-poly <vilib>:"WPI_SwitchOpen.vi"("Normally Closed"=w126, "DIO Channel"=w127) -> ("error out"=w125:errorcluster, "SwitchDevRef"=w124:T40)  [unwired: 8 in]
          n64 = call <vilib>:"WPI_SwitchRefNum Registry Set.vi"("error in (no error)"=w125, "refnum name"=w123, "SwitchDevRef"=w124) -> ("error out"=w121:errorcluster, "SwitchDevRef"=w122:T40)  [unwired: 7 in]
        }
      }
    }
  }
  n65 = in-place {
    in-place-border: "HARDWARE cluster" -> [w131]
    in-place-border: [w129] -> w9
    # "define SONARS"
    n66 = Unbundle By Name(w131) -> ("SONAR"=w130:T26[])
    n67 = for {
      tunnel: w130 -> [w133] mode=indexing
      tunnel: [w132] -> w129
      n68 = disable-structure shown="Disabled" {
        disable-tunnel: w133 -> [w135 _]
        disable-tunnel: [w134 _] -> w132
        frame Disabled {
          n69 = Unbundle By Name(w135) -> ("Installed?"=w136:bool)
          n70 = case shown="True" w136 {
            tunnel: w135 -> [_ w142]
            tunnel: [_ w137] -> w134
            frame False {
            }
            frame True {
              n71 = Unbundle By Name(w142) -> ("Device type"=w139:T27, "PING Channel"=w141:T6, "ECHO Channel"=w140:T6, "RefName"=w138:string)  [unwired: 2 out]
              n72 = case shown="\"SRF08 Digital\"" w139 {
                tunnel: w141 -> [w148 w153 _ _]
                tunnel: w140 -> [w147 _ _ _]
                tunnel: w138 -> [w145 w149 w154 w162]
                tunnel: [w143 w151 w157 w164] -> w137
                frame "SRF04 Digital", Default {
                  n73 = call-poly <vilib>:"WPI_UltrasonicOpen.vi"("Echo DIO Channel"=w147, "Ping DIO Channel"=w148) -> ("error out"=w146:errorcluster, "SonarSRF04DevRef"=w144:T43)  [unwired: 8 in]
                  n74 = call-poly <vilib>:"WPI_UltrasonicRefNum Registry Set.vi"("error in (no error)"=w146, "refnum name"=w145, "SonarSRF04DevRef"=w144) -> ("error out"=w143:errorcluster)  [unwired: 7 in, 1 out]
                }
                frame "MB1010 Digital" {
                  n75 = call-poly <vilib>:"WPI_UltrasonicOpen.vi"("Ping DIO Channel"=w153) -> ("error out"=w152:errorcluster, "SonarSRF04DevRef"=w150:T43)  [unwired: 9 in]
                  n76 = call-poly <vilib>:"WPI_UltrasonicRefNum Registry Set.vi"("error in (no error)"=w152, "refnum name"=w149, "SonarSRF04DevRef"=w150) -> ("error out"=w151:errorcluster)  [unwired: 7 in, 1 out]
                }
                frame "MB1010 Analog" {
                  n77 = call-poly <vilib>:"WPI_UltrasonicOpen.vi"("error in (no error)"=errorcluster {"status"=FALSE, "code"=0, "source"=""} ("error in"), "Echo DIO Channel"=u8 3 ("Average Bits"), 10:0.0098 ("Scaling factor (V/in)"), "Ping DIO Channel"=FPGA_AIChannel."AI 0" ("Analog Channel")) -> ("error out"=w156:errorcluster, "SonarSRF04DevRef"=w155:T43)  [unwired: 6 in]
                  n78 = call-poly <vilib>:"WPI_UltrasonicRefNum Registry Set.vi"("error in (no error)"=w156, "refnum name"=w154, "SonarSRF04DevRef"=w155) -> ("error out"=w157:errorcluster)  [unwired: 7 in, 1 out]
                }
                frame "SRF08 Digital" {
                  w167 = T44 224 items=["Dev 0"=224, "Dev 1"=226, "Dev 2"=228, "Dev 3"=230, "Dev 4"=232, "Dev 5"=234, "Dev 6"=236, "Dev 7"=238, "Dev 8"=240, "Dev 9"=242, "Dev 10"=244, "Dev 11"=246, "Dev 12"=248, "Dev 13"=250, "Dev 14"=252, "Dev 15"=254] ("Device Address")
                  n79 = call-poly <vilib>:"WPI_UltrasonicOpen.vi"("error in (no error)"=errorcluster {"status"=FALSE, "code"=0, "source"=""} ("error in"), 10:w167, "Ping DIO Channel"=i2c_bus."I2C On-Board" ("I2C Bus")) -> ("error out"=w163:errorcluster, "SonarSRF04DevRef"=w165:T43)  [unwired: 7 in]
                  n80 = call-poly <vilib>:"WPI_UltrasonicRefNum Registry Set.vi"("error in (no error)"=w163, "refnum name"=w162, "SonarSRF04DevRef"=w165) -> ("error out"=w164:errorcluster)  [unwired: 7 in, 1 out]
                }
              }
            }
          }
        }
        frame Enabled {
        }
      }
    }
  }
  n81 = in-place {
    in-place-border: "HARDWARE cluster" -> [w172]
    in-place-border: [w170] -> _
    in-place-border: [w169] -> w11
    # "define SERVOS"
    n82 = Unbundle By Name(w172) -> ("SERVOS"=w171:T25[])
    n83 = for {
      tunnel: w171 -> [w175] mode=indexing
      tunnel: [w174] -> w170
      tunnel: [w173] -> w169
      n84 = Unbundle By Name(w175) -> ("Installed?"=w176:bool)
      n85 = case shown="True" w176 {
        tunnel: w175 -> [_ w184]
        tunnel: [_ w178] -> w174
        tunnel: [_ w177] -> w173
        frame False {
        }
        frame True {
          n86 = Unbundle By Name(w184) -> ("PWM ch"=w180:T4, "Angular range"=w179:dbl, "RefName"=w181:string)
          n87 = call <vilib>:"WPI_ServoOpen.vi"("Angular Range"=w179, "PWM Channel"=w180) -> ("error out"=w183:errorcluster, "ServoDeviceRef"=w182:T45)  [unwired: 8 in]
          n88 = call <vilib>:"WPI_ServoRefNum Registry Set.vi"("error in (no error)"=w183, "refnum name"=w181, "ServoDeviceRef"=w182) -> ("error out"=w177:errorcluster, "ServoDeviceRef"=w178:T45)  [unwired: 7 in]
        }
      }
    }
  }
  n89 = in-place {
    in-place-border: "HARDWARE cluster" -> [w188]
    in-place-border: [w186] -> _
    in-place-border: [w185] -> w10
    # "define GYRO"
    n90 = Unbundle By Name(w188) -> ("GYRO HARDWARE"=w187:T16)
    n91 = disable-structure shown="Disabled" {
      disable-tunnel: w187 -> [w191 _]
      disable-tunnel: [w190 _] -> w186
      disable-tunnel: [w189 _] -> w185
      frame Disabled {
        n92 = Unbundle By Name(w191) -> ("Installed?"=w192:bool)
        n93 = case shown="True" w192 {
          tunnel: w191 -> [_ w206]
          tunnel: [_ w197] -> w190
          tunnel: [_ w196] -> w189
          frame False {
          }
          frame True {
            n94 = Unbundle By Name(w206) -> ("SPI Bus"=w205:T17, "AnalogChannel"=w200:T18, "Calibrate On Open"=w202:bool, "Calibrated Center Voltage"=w201:dbl, "Calibration Time (s)"=w204:dbl, "Sample Rate (Hz)"=w203:dbl, "RefName"=w193:string)
            n95 = case shown="Default" w205 {
              selector: w205 -> [_ w219]
              tunnel: w204 -> [w207 w218]
              tunnel: w203 -> [_ w217]
              tunnel: w202 -> [w208 w216]
              tunnel: w201 -> [w209 w215]
              tunnel: [w212 w214] -> w195
              tunnel: [w211 w213] -> w194
              tunnel: w200 -> [w210 _]
              frame "Invalid" {
                n96 = call-poly <vilib>:"WPI_GyroOpen.vi"("Calibrated Center Voltage"=w209, "Calibration Time (s)"=w207, "Calibrate On Open"=w208, "Analog Channel"=w210) -> ("error out"=w211:errorcluster, "GyroDevRef"=w212:T46)  [unwired: 5 in, 1 out]
              }
              frame Default {
                n97 = call-poly <vilib>:"WPI_GyroOpen.vi"("Calibrated Center Voltage"=w215, "Calibration Time (s)"=w218, "Calibrate On Open"=w216, "Analog Channel"=w217, 11:w219) -> ("error out"=w213:errorcluster, "GyroDevRef"=w214:T46)  [unwired: 4 in, 1 out]
              }
            }
            n98 = call <vilib>:"WPI_GyroRefNum Registry Set.vi"("error in (no error)"=w194, "refnum name"=w193, "GyroDevRef"=w195) -> ("error out"=w199:errorcluster, "GyroDevRef"=w198:T46)  [unwired: 7 in]
            n99 = call <vilib>:"WPI_GyroReset.vi"("error in"=w199, "GyroDevRef"=w198) -> ("error out"=w196:errorcluster, "GyroDevRef"=w197:T46)  [unwired: 8 in]
          }
        }
      }
      frame Enabled {
      }
    }
  }
  n100 = in-place {
    in-place-border: "HARDWARE cluster" -> [w223]
    in-place-border: [w221] -> _
    in-place-border: [w220] -> w4
    # "define INPUT CONTROLLERS"
    n101 = Unbundle By Name(w223) -> ("Controller"=w222:T11[])
    n102 = for {
      tunnel: w222 -> [w226] mode=indexing
      tunnel: [w225] -> w221
      tunnel: [w224] -> w220
      n103 = Unbundle By Name(w226) -> ("Installed?"=w227:bool)
      n104 = case shown="True" w227 {
        tunnel: w226 -> [_ w233]
        tunnel: [_ w229] -> w225
        tunnel: [_ w228] -> w224
        frame False {
        }
        frame True {
          n105 = Unbundle By Name(w233) -> ("RefName"=w230:string, "JoystickDevice"=w232:T12)
          n106 = call <vilib>:"WPI_JoystickOpen.vi"("JoystickDevice"=w232) -> ("JoystickDevRef"=w231:T47)  [unwired: 10 in]
          n107 = call <vilib>:"WPI_JoystickRefNum Registry Set.vi"("refnum name"=w230, "JoystickDevRef"=w231) -> ("error out"=w228:errorcluster, "JoystickDevRef"=w229:T47)  [unwired: 8 in]
        }
      }
    }
  }
  n108 = Merge Errors(w13, w12, w3) -> (w8:errorcluster)
  n109 = in-place {
    in-place-border: "HARDWARE cluster" -> [w240]
    in-place-border: [w239] -> w7
    # "REVISED to use SPARK MAX by TDM 20-01-26"
    # "define DRIVE SYSTEM MOTORS"
    n110 = in-place {
      in-place-border: w240 -> [w269]
      in-place-border: [w258] -> w238
      in-place-border: [w246] -> w235
      in-place-border: [w244] -> w234
      n111 = Unbundle By Name(w269) -> ("DRIVE MOTORS"=w248:T8[])
      n112 = Index Array(array=w248, index #1=0 ("index")) -> (element #1=w267:T8, element #2=w266:T8)  [unwired: 1 in]
      n113 = Index Array(array=w248, index #1=2 ("index")) -> (element #1=w256:T8, element #2=w255:T8)  [unwired: 1 in]
      n114 = Unbundle By Name(w267) -> ("RefName"=w246:string, "Installed?"=w265:bool, "CAN ID"=w261:u8, "Invert?"=w260:bool)  [unwired: 1 out]
      n115 = Unbundle By Name(w266) -> ("Installed?"=w263:bool, "CAN ID"=w262:u8)  [unwired: 2 out]
      n116 = Unbundle By Name(w256) -> ("Installed?"=w254:bool, "CAN ID"=w250:u8, "Invert?"=w249:bool)  [unwired: 1 out]
      n117 = Unbundle By Name(w255) -> ("Installed?"=w252:bool, "CAN ID"=w251:u8)  [unwired: 2 out]
      n118 = And(x=w265, y=w263) -> (x .and. y?=w264:bool)
      n119 = And(x=w254, y=w252) -> (x .and. y?=w253:bool)
      n120 = case shown="True" w264 {
        tunnel: w261 -> [_ w283]
        tunnel: w262 -> [_ w282]
        tunnel: w260 -> [_ w281]
        tunnel: [_ w280] -> w259
        tunnel: [_ w279] -> w243
        tunnel: [_ w278] -> w242
        frame False {
        }
        frame True {
          n121 = call <vilib>:"Spark MAX Open.vi"("Invert"=w281, "Device Number"=w283) -> ("error out"=w279:errorcluster, "MotorControlDeviceRef"=w280:T2)  [unwired: 8 in]
          n122 = call <vilib>:"Spark MAX Open.vi"("Device Number"=w282) -> ("error out"=w285:errorcluster, "MotorControlDeviceRef"=w284:T2)  [unwired: 9 in]
          n123 = call <vilib>:"Spark MAX Follow.vi"("error in (no error)"=w285, "Master Controller"=w280, "MotorControlDeviceRef"=w284) -> ("error out"=w278:errorcluster)  [unwired: 7 in, 1 out]
        }
      }
      n124 = case shown="True" w253 {
        tunnel: w250 -> [_ w275]
        tunnel: w251 -> [_ w274]
        tunnel: w249 -> [_ w273]
        tunnel: [_ w272] -> w247
        tunnel: [_ w271] -> w245
        tunnel: [_ w270] -> w241
        frame False {
        }
        frame True {
          n125 = call <vilib>:"Spark MAX Open.vi"("Invert"=w273, "Device Number"=w275) -> ("error out"=w270:errorcluster, "MotorControlDeviceRef"=w272:T2)  [unwired: 8 in]
          n126 = call <vilib>:"Spark MAX Open.vi"("Device Number"=w274) -> ("error out"=w277:errorcluster, "MotorControlDeviceRef"=w276:T2)  [unwired: 9 in]
          n127 = call <vilib>:"Spark MAX Follow.vi"("error in (no error)"=w277, "Master Controller"=w272, "MotorControlDeviceRef"=w276) -> ("error out"=w271:errorcluster)  [unwired: 7 in, 1 out]
        }
      }
      n128 = Build Array(w259, w247) -> (w258:T2[])
      n129 = Merge Errors(w243, w242, w241, w245) -> (w244:errorcluster)
    }
    n130 = in-place {
      in-place-border: w238 -> [w295]
      in-place-border: [w289] -> w237
      in-place-border: [w288] -> w236
      in-place-border: w234 -> [w287]
      n131 = Bundle By Name(cluster=T1 {"DevStatus"={"status"=FALSE, "code"=0, "source"=""}, "Motors[]"=[], "Square Inputs"=FALSE, "Max Output"=1.0} ("RobotDriveDevRef"), "Max Output"=1.0, "Square Inputs"=TRUE, "Motors[]"=w295, "DevStatus"=w287) -> (w293:T1)
      n132 = call <vilib>:"WPI_RobotDriveSafetyConfig.vi"("error in (no error)"=w287, "timeout (s)"=0.1, "mode"=WPI_SafetyOutputConfigMenu."Enable", "RobotDriveDevRef"=w293) -> ("error out"=w288:errorcluster, "RobotDriveDevRef"=w289:T1)  [unwired: 6 out]
    }
    "RobotDriveDevRef" <- w237
    n133 = in-place {
      in-place-border: [w303] -> w239
      in-place-border: w237 -> [w302]
      in-place-border: w236 -> [w301]
      in-place-border: w235 -> [w300]
      n134 = call <vilib>:"WPI_RobotDriveRefNum Registry Set.vi"("error in (no error)"=w301, "refnum name"=w300, "RobotDriveDevRef"=w302) -> ("error out"=w297:errorcluster, "RobotDriveDevRef"=w299:T1)  [unwired: 1 in, 6 out]
      n135 = call <vilib>:"WPI_RobotDriveSafetyConfig.vi"("error in (no error)"=w297, "timeout (s)"=0.5, "mode"=WPI_SafetyOutputConfigMenu."Enable", "RobotDriveDevRef"=w299) -> ("error out"=w303:errorcluster)  [unwired: 6 in, 1 out]
    }
  }
  n136 = in-place {
    in-place-border: "HARDWARE cluster" -> [w307]
    in-place-border: [w305] -> _
    in-place-border: [w304] -> w5
    # "define ENCODERS"
    n137 = Unbundle By Name(w307) -> ("ENCODERS"=w306:T14[])
    n138 = for {
      tunnel: w306 -> [w310] mode=indexing
      tunnel: [w309] -> w305
      tunnel: [w308] -> w304
      n139 = Unbundle By Name(w310) -> ("Installed?"=w311:bool)
      n140 = case shown="True" w311 {
        tunnel: w310 -> [_ w335]
        tunnel: [_ w319] -> w309
        tunnel: [_ w320] -> w308
        frame False {
        }
        frame True {
          n141 = Unbundle By Name(w335) -> ("A Channel"=w330:T6, "B Channel"=w329:T6, "Invert Direction"=w327:bool, "Enum"=w328:T15, "Gear ratio"=w318:dbl, "Cycles per Rev"=w322:dbl, "Diameter (in)"=w323:dbl[unit], "RefName"=w324:string, "min rate (hz)"=w313:dbl, "Samples"=w312:u8)
          n142 = in-place {
            in-place-border: w323 -> [w343]
            in-place-border: w322 -> [w340]
            in-place-border: [w339] -> w321
            in-place-border: w318 -> [w336]
            n143 = node(w343) -> (w342:dbl)
            n144 = Multiply(x=3.141592653589793, y=w342) -> (x*y=w337:dbl)
            n145 = Divide(x=w337, y=w336) -> (x/y=w338:dbl)
            n146 = Divide(x=w338, y=w340) -> (x/y=w339:dbl)
          }
          n147 = call <vilib>:"WPI_DigitalInputOpen.vi"("DIO Channel"=w330) -> ("DigitalInputDevRef"=w332:T49)  [unwired: 1 in, 9 out]
          n148 = call <vilib>:"WPI_DigitalInputOpen.vi"("DIO Channel"=w329) -> ("DigitalInputDevRef"=w333:T49)  [unwired: 1 in, 9 out]
          n149 = call-poly <vilib>:"WPI_CounterToDigitalSource.vi"("DigitalInputDevRef"=w332) -> ("Digital Source"=w331:T50)  [unwired: 6 out]
          n150 = call-poly <vilib>:"WPI_CounterToDigitalSource.vi"("DigitalInputDevRef"=w333) -> ("Digital Source"=w334:T50)  [unwired: 6 out]
          n151 = call <vilib>:"WPI_EncoderOpen.vi"("DistancePerCount"=w321, "Decoding Type"=w328, "Invert Direction (False)"=w327, "BSource"=w334, "ASource"=w331) -> ("error out"=w326:errorcluster, "EncoderDevRef"=w325:T54)  [unwired: 3 in, 2 out]
          n152 = call <vilib>:"WPI_EncoderRefNum Registry Set.vi"("error in (no error)"=w326, "refnum name"=w324, "EncoderDevRef"=w325) -> ("error out"=w316:errorcluster, "EncoderDevRef"=w317:T54)  [unwired: 7 in]
          n153 = call <vilib>:"WPI_EncoderConfigureTimer.vi"("error in (no error)"=w316, "Number Samples to Average"=w312, "Minimum Rate"=w313, "EncoderDevRef"=w317) -> ("error out"=w314:errorcluster, "EncoderDevRef"=w315:T54)  [unwired: 6 in]
          n154 = call <vilib>:"WPI_EncoderReset.vi"("error in (no error)"=w314, "EncoderDevRef"=w315) -> ("error out"=w320:errorcluster, "EncoderDevRef"=w319:T54)  [unwired: 8 in]
        }
      }
    }
  }
  n155 = in-place {
    in-place-border: "HARDWARE cluster" -> [w346]
    in-place-border: [w344] -> w6
    # "define MOTORS (not in drive system)"
    n156 = Unbundle By Name(w346) -> ("MOTORS"=w345:T8[])
    n157 = for {
      tunnel: w345 -> [w348] mode=indexing
      tunnel: [w349] -> w344
      tunnel: [w347] -> _
      n158 = Unbundle By Name(w348) -> ("Motor Controller"=w351:T9, "Installed?"=w350:bool)
      n159 = case shown="True" w350 {
        tunnel: w351 -> [_ w361]
        tunnel: [_ w358] -> w349
        tunnel: w348 -> [_ w357]
        tunnel: [_ w352] -> w347
        frame False {
        }
        frame True {
          n160 = Unbundle By Name(w357) -> ("PWM ch"=w356:T4, "Invert?"=w355:bool, "remove deadband"=w354:bool, "RefName"=w353:string)
          n161 = case shown="7" w361 {
            tunnel: [w366 w371 w376 w381 w386 w391 w396] -> w360
            tunnel: [w365 w370 w375 w380 w385 w390 w395] -> w359
            tunnel: w356 -> [w364 w369 w374 w379 w384 w389 w394]
            tunnel: w354 -> [w363 w368 w373 w378 w383 w388 w393]
            tunnel: w355 -> [w362 w367 w372 w377 w382 w387 w392]
            frame 0, Default {
              n162 = call-poly <vilib>:"WPI_MotorControlOpen.vi"("Invert"=w362, "Eliminate Deadband"=w363, "PWM Channel"=w364) -> ("error out"=w365:errorcluster, "MotorControlDeviceRef"=w366:T2)  [unwired: 7 in]
            }
            frame 2 {
              n163 = call-poly <vilib>:"WPI_MotorControlOpen.vi"("Invert"=w367, "Eliminate Deadband"=w368, "PWM Channel"=w369) -> ("error out"=w370:errorcluster, "MotorControlDeviceRef"=w371:T2)  [unwired: 7 in]
            }
            frame 3 {
              n164 = call-poly <vilib>:"WPI_MotorControlOpen.vi"("Invert"=w372, "Eliminate Deadband"=w373, "PWM Channel"=w374) -> ("error out"=w375:errorcluster, "MotorControlDeviceRef"=w376:T2)  [unwired: 7 in]
            }
            frame 4 {
              n165 = call-poly <vilib>:"WPI_MotorControlOpen.vi"("Invert"=w377, "Eliminate Deadband"=w378, "PWM Channel"=w379) -> ("error out"=w380:errorcluster, "MotorControlDeviceRef"=w381:T2)  [unwired: 7 in]
            }
            frame 5 {
              n166 = call-poly <vilib>:"WPI_MotorControlOpen.vi"("Invert"=w382, "Eliminate Deadband"=w383, "PWM Channel"=w384) -> ("error out"=w385:errorcluster, "MotorControlDeviceRef"=w386:T2)  [unwired: 7 in]
            }
            frame 6 {
              n167 = call-poly <vilib>:"WPI_MotorControlOpen.vi"("Invert"=w387, "Eliminate Deadband"=w388, "PWM Channel"=w389) -> ("error out"=w390:errorcluster, "MotorControlDeviceRef"=w391:T2)  [unwired: 7 in]
            }
            frame 7 {
              n168 = call-poly <vilib>:"WPI_MotorControlOpen.vi"("Invert"=w392, "Eliminate Deadband"=w393, "PWM Channel"=w394) -> ("error out"=w395:errorcluster, "MotorControlDeviceRef"=w396:T2)  [unwired: 7 in]
            }
          }
          n169 = call <vilib>:"WPI_MotorControlRefNum Registry Set.vi"("error in (no error)"=w359, "refnum name"=w353, "MotorControlDevRef"=w360) -> ("error out"=w358:errorcluster, "MotorControlDevRef"=w352:T2)  [unwired: 7 in]
        }
      }
    }
  }
  n170 = Merge Errors(w4, w10, w11, w9, w8) -> (w2:errorcluster)
  n171 = Merge Errors(w7, w6, w5, w2) -> (→"error out":errorcluster)
